vi "attendedmode.vi"() -> ()   [LabVIEW 2017]
panel:
  in  "Numeric":dbl
  out "error out":errorcluster
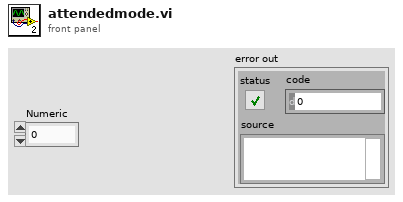
[diagram p1: front panel]
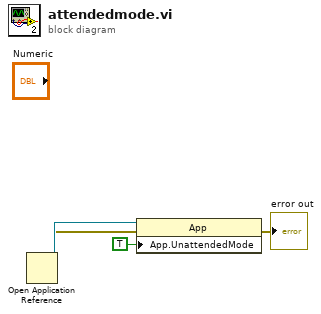
[diagram p0: block diagram]
diagram:
  n1 = Open Application Reference() -> (0:w3:errorcluster, 3:w4:refnum<vi>)  [unwired: 4 in]
  n2 = property class="App"(reference=w4, error in=w3, "App.UnattendedMode"=TRUE ("Application:Unattended Mode")) -> (error out=→"error out":errorcluster)  [unwired: 1 out]
